vi "RT_control.vi"() -> ()   [LabVIEW 2019]
uses:
  <vilib>/platform/TimedLoop/XDataNode/XDataNode.xnode
  <vilib>/Platform/TimedLoop/XDataNode/nitl_modes.ctl
  <vilib>/Platform/TimedLoop/XDataNode/XDNodeRunTimeDep.lvlib
  <vilib>/Platform/TimedLoop/XDataNode/wakeup.ctl
  <vilib>/Platform/TimedLoop/XDataNode/timing_clust.ctl
  <vilib>/Utility/file.llb/Write Delimited Spreadsheet (DBL).vi
  <vilib>/myRIO/Instrument Drivers/Onboard IO/PWM/PWM.lvlib
  <vilib>/Utility/Variable/NI_VariableUtilities.lvlib
  <vilib>/myRIO/Express VI/IRQ/IRQ Express VI.xnode
  rpm.vi
  <vilib>/myRIO/Instrument Drivers/IRQ/IO IRQ/IO IRQ.lvlib
  <vilib>/myRIO/Common/Instrument Driver Framework/myRIO v1.0/IRQ/typedefs/DI IRQ Type.ctl
  ISR.vi
  <vilib>/myRIO/Common/Instrument Driver Framework/myRIO v1.0/IRQ/typedefs/Callback VI Ref.ctl
  <vilib>/myRIO/Instrument Drivers/IRQ/IO IRQ/vis/myRIO Register DI IRQ.xnode
  <vilib>/myRIO/Common/Instrument Driver Framework/myRIO v1.0/IRQ/vis/myRIO v1.1 Register DI IRQ.vi
  <vilib>/userDefined/High Color/nirio_resource_hc.ctl
  <vilib>/Analysis/NI_AALBase.lvlib
panel:
  out "tf":dbl
  out "fs":dbl
  out "N":i32
  out "i":i32
  out "Max. Iteration Duration":i64
  out "error out (no error) 2":errorcluster
  out "Iteration Duration":i64
  out "omega_vec":dbl[](array[numeric])
  out "Interrupt On":bool
  in  "RPM Inst Data":path=path "/tmp/log.csv"
  out "Omega":dbl[](graph)
  in  "error in (no error)":errorcluster
  out "Np":dbl
  out "ft":dbl
  in  "Input Data":path=path "/tmp/log.csv"
  out "Finished late":bool
  out "Acquisition State":bool
  in  "Run Time (s)":dbl
  in  "Sampling \nFrequency (Hz)":dbl
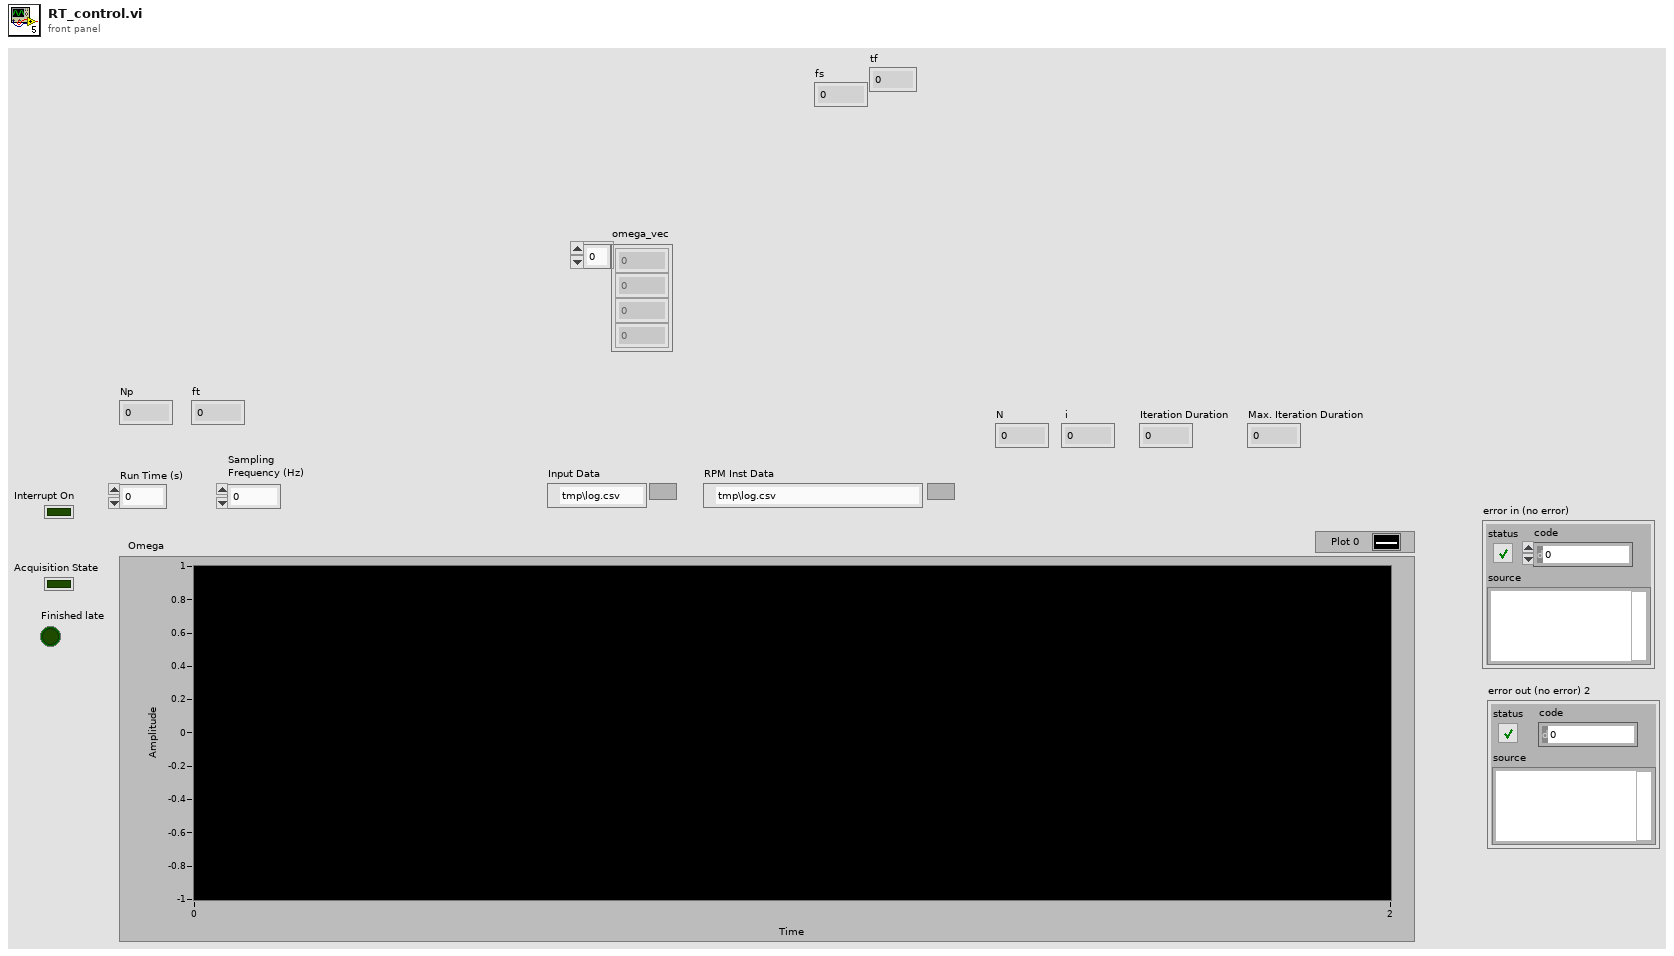
[diagram p1: front panel]
types:
  T1 = typedef "PWM.lvlib/PWM Reference.ctl" = cluster{"myRIO Reference":T2, "PWM Channels Enum":T6, "PWM Configuration":T7}
  T2 = typedef "myRIO Generic Hardware Reference.ctl" = cluster{"myRIO Model":T3, "myRIO Hardware Reference":T4}
  T3 = typedef "Hardware Version Enum.ctl" = enum16{"Unknown", "myRIO-1900", "myRIO-1950", "roboRIO", "NI ELVIS RIO CM", "ELVIS III"}
  T4 = typedef "myRIO v1.0 Reference.ctl" = cluster{"Generic FPGA Reference":T5, "Allow multiple opens":bool}
  T5 = typedef "Generic FPGA Reference.ctl" = refnum<k20>
  T6 = typedef "PWM Channels Enum.ctl" = enum16{"Not Connected", "C/PWM0", "C/PWM1", "A/PWM0", "A/PWM1", "A/PWM2", "A/PWM3", "A/PWM4", "A/PWM5", "A/PWM6", "A/PWM7", "A/PWM8", "A/PWM9", "A/PWM10", "A/PWM11", "A/PWM12", "A/PWM13", "A/PWM14", "A/PWM15", "A/PWM16", "A/PWM17", "A/PWM18", "A/PWM19", "B/PWM0", "B/PWM1", "B/PWM2", "B/PWM3", "B/PWM4", "B/PWM5", "B/PWM6", "B/PWM7", "B/PWM8", "B/PWM9", "B/PWM10", "B/PWM11", "B/PWM12", "B/PWM13", "B/PWM14", "B/PWM15", "B/PWM16", "B/PWM17", "B/PWM18", "B/PWM19", "PWM/PWM0", "PWM/PWM1", "PWM/PWM2", "PWM/PWM3", "PWM/PWM4", "PWM/PWM5", "PWM/PWM6", "PWM/PWM7", "PWM/PWM8", "PWM/PWM9"}
  T7 = typedef "PWM.lvlib/PWM Configuration.ctl" = cluster{"Frequency":dbl, "Duty Cycle":dbl}
  T8 = typedef "XDNodeRunTimeDep.lvlib/timing_clust.ctl" = cluster{"Expected End [f-1]":u64, "Actual End [f-1]":u64, "Finished Late? [f-1]":bool, "Expected End [i-1]":u64, "Actual End [i-1]":u64, "Finished Late? [i-1]":bool, "Expected Start [i]":u64, "Actual Start [i]":u64, "Expected Start [f]":u64, "Actual Start [f]":u64, "Source Name":string, "Structure Name":string, "Period":i64, "Deadline":i64, "Offset":i64, "Start":i64, "Priority":i32, "Timeout":i32, "Mode":T9, "Wakeup Reason":T10, "Error":errorcluster, "Source Type":string, "Secondary Source Type":string, "Global End Time":u64, "Global Start Time":u64, "Frame Duration":u64, "Iteration Duration":u64, "Assigned CPU":i32, "I/O Scan Engine Mode":u32}
  T9 = typedef "XDNodeRunTimeDep.lvlib/nitl_modes.ctl" = enum32{"No Change", "Process missed periods, maintain original phase", "Discard missed periods, maintain original phase", "Process missed periods, ignore original phase", "Discard missed periods, ignore original phase"}
  T10 = typedef "XDNodeRunTimeDep.lvlib/wakeup.ctl" = enum32{"Normal", "Aborted", "Asynchronous wakeup", "Timing source error", "Timed loop error", "Timeout"}
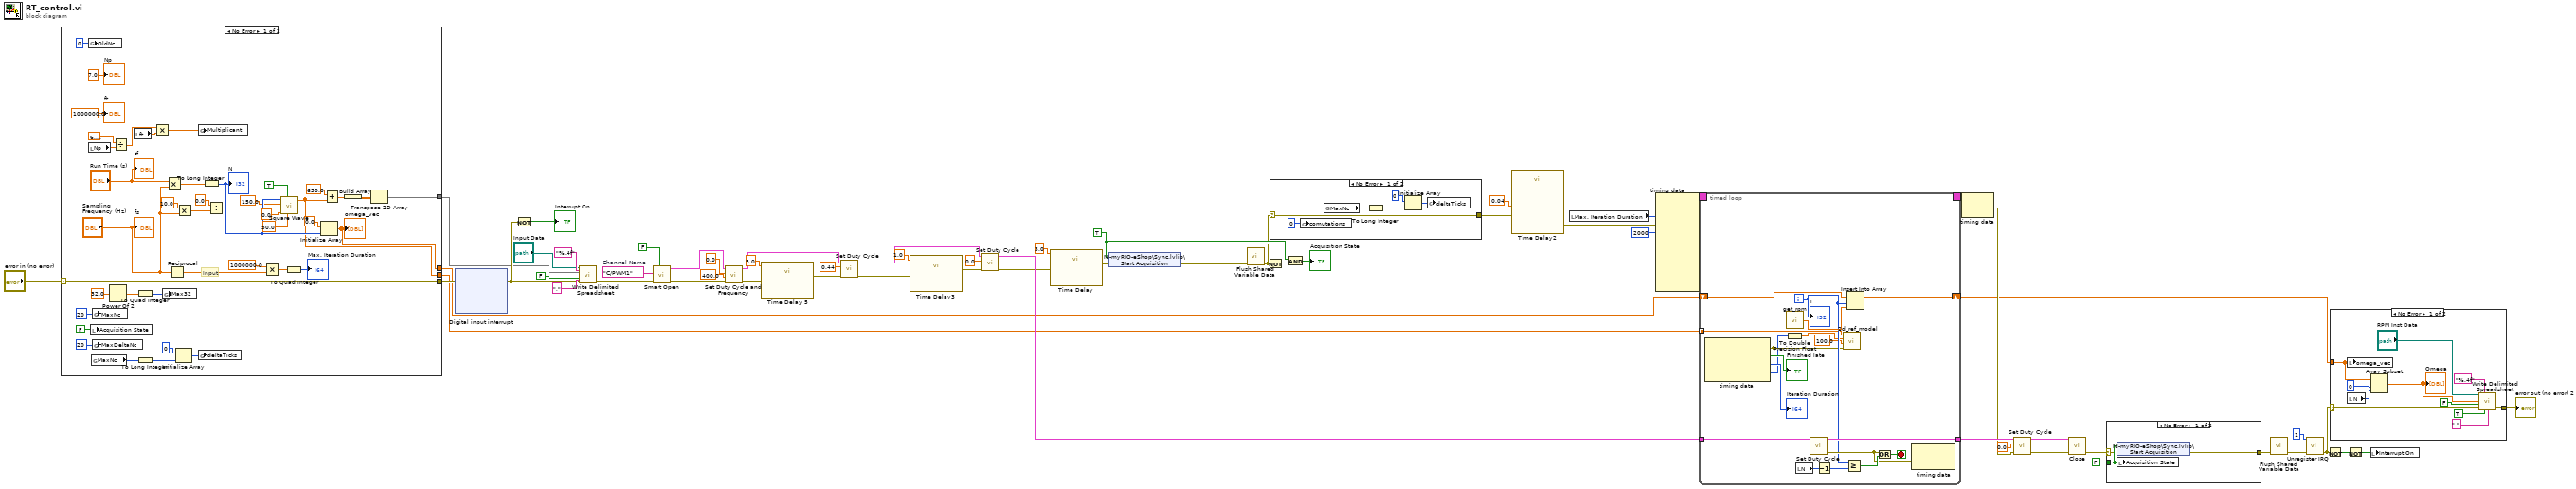
[diagram p0: block diagram]
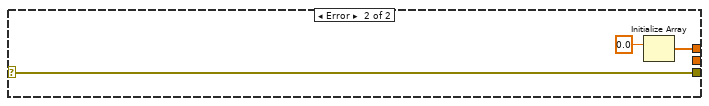
[diagram p5: hidden frame]
diagram:
  w54 = tag "C/PWM1"  # Channel Name
  w37 = TRUE ("Acquisition State")
  n1 = case shown="No Error" "error in (no error)" {
    selector: "error in (no error)" -> [w98 w104]
    tunnel: [w98 w104] -> w34
    tunnel: [w81 w102] -> w9
    tunnel: [w79 _] -> w2
    tunnel: [w60 _] -> w1
    frame No Error {
      # "Input"
      n2 = local read "Np"() -> (w94:dbl)
      n3 = global write "rpm.vi" "OldNc"(i64 0 ("MaxNc")) -> ()
      n4 = local write "Acquisition State"(FALSE ("Acquisition State")) -> ()
      n5 = global read "rpm.vi" "MaxNc"() -> (w83:i64)
      n6 = global write "rpm.vi" "MaxNc"(i64 20 ("MaxNc")) -> ()
      n7 = global write "rpm.vi" "MaxDeltaNc"(i64 20 ("MaxDeltaNc")) -> ()
      n8 = Power Of 2(x=32.0) -> (2^x=w100:dbl)
      n9 = Divide(x=6.283185307179586, y=w94) -> (x/y=w93:dbl)
      n10 = local read "ft"() -> (w92:dbl)
      n11 = To Quad Integer(1:w100) -> (0:w91:i64)
      n12 = To Long Integer(number=w83) -> (32bit integer=w82:i32)
      n13 = Multiply(x=w93, y=w92) -> (x*y=w101:dbl)
      n14 = global write "rpm.vi" "Max32"(w91) -> ()
      n15 = Multiply(x="Run Time (s)", y="Sampling \nFrequency (Hz)") -> (x*y=w75:dbl)
      n16 = Reciprocal(x="Sampling \nFrequency (Hz)") -> (1/x=w78:dbl)
      n17 = Initialize Array(i64 0, w82) -> (w84:i64[])
      n18 = Multiply(x=10.0, y="Sampling \nFrequency (Hz)") -> (x*y=w63:dbl)
      n19 = global write "rpm.vi" "Multiplicant"(w101) -> ()
      n20 = global write "rpm.vi" "deltaTicks"(w84) -> ()
      n21 = To Long Integer(number=w75) -> (32bit integer=w72:i32)
      "N" <- w72
      n22 = Divide(x=0.0, y=w63) -> (x/y=w65:dbl)
      n23 = Multiply(x=1000000.0, y=w78) -> (x*y=w76:dbl)
      n24 = call <vilib>:"Square Wave.vi"("samples"=w72, "reset phase"=TRUE, "amplitude"=150.0, "frequency"=w65, "duty cycle (%)"=50.0, "phase in"=0.0) -> ("square wave"=w60:dbl[])  [unwired: 2 out]
      n25 = To Quad Integer(1:w76) -> (0:→"Max. Iteration Duration":i64)
      n26 = Initialize Array(0.0 ("element"), w72) -> (w81:dbl[])
      "omega_vec" <- w81
      n27 = Add(x=650.0, y=w60) -> (x+y=w67:dbl[])
      n28 = Build Array(w67) -> (w80:dbl[][])
      n29 = Transpose 2D Array(2D array=w80) -> (transposed array=w79:dbl[][])
      "Np" <- 7.0 ("Numeric")
      "ft" <- 1000000.0 ("ft")
      "fs" <- "Sampling \nFrequency (Hz)"
      "tf" <- "Run Time (s)"
    }
    frame Error {
      n30 = Initialize Array(0.0 ("element")) -> (w102:dbl[])  [unwired: 1 in]
    }
  }
  n31 = xnode "Digital input interrupt"("error in (no error)"=w34) -> ("error out"=w29:errorcluster)
  n32 = Not(x=w29) -> (.not. x?=→"Interrupt On":bool)
  n33 = call-poly <vilib>:"Write Delimited Spreadsheet.vi"("file path (dialog if empty)"="Input Data", "format (%.3f)"="%.4f", "2D data"=w2, "append to file? (new file:F)"=FALSE, "error in (no error)"=w29, "delimiter (\\t)"="," ("delimiter (\\t)")) -> ("error out"=w50:errorcluster)  [unwired: 8 in, 1 out]
  n34 = call <vilib>:"Smart Open.vi"("Allow multiple opens?"=FALSE, "error in (no error)"=w50, "Channel Name"=w54) -> ("error out"=w52:errorcluster, "PWM Ref Out"=w53:T1)  [unwired: 7 in]
  n35 = call <vilib>:"Set Duty Cycle and Frequency.vi"("error in (no error)"=w52, "Frequency [Hz]"=400.0, "Duty Cycle"=0.0, "PWM Ref In"=w53) -> ("error out"=w27:errorcluster, "PWM Ref Out"=w17:T1)  [unwired: 5 in]
  n36 = call "Time Delay 5"("error in (no error)"=w27, "Delay Time (s)"=5.0) -> ("error out"=w18:errorcluster)  [unwired: 9 in]
  n37 = call <vilib>:"Set Duty Cycle.vi"("error in (no error)"=w18, "Duty Cycle"=0.44, "PWM Ref In"=w17) -> ("error out"=w21:errorcluster, "PWM Ref Out"=w15:T1)  [unwired: 6 in]
  n38 = call "Time Delay3"("error in (no error)"=w21, "Delay Time (s)"=1.0) -> ("error out"=w16:errorcluster)  [unwired: 9 in]
  n39 = call <vilib>:"Set Duty Cycle.vi"("error in (no error)"=w16, "Duty Cycle"=0.0, "PWM Ref In"=w15) -> ("error out"=w25:errorcluster, "PWM Ref Out"=w26:T1)  [unwired: 6 in]
  n40 = call "Time Delay"("error in (no error)"=w25, "Delay Time (s)"=3.0) -> ("error out"=w45:errorcluster)  [unwired: 9 in]
  n41 = shared-variable "NI-myRIO-eShop\\Sync.lvlib\\Start Acquisition"(w37, error in=w45) -> (error out=w49:errorcluster)
  n42 = call <vilib>:"Flush Shared Variable Data.vi"("error in (no error)"=w49) -> ("error out"=w23:errorcluster)  [unwired: 10 in]
  n43 = Not(x=w23) -> (.not. x?=w22:bool)
  n44 = case shown="No Error" w23 {
    selector: w23 -> [w109 w111]
    tunnel: [w109 w111] -> w31
    frame No Error {
      n45 = global write "rpm.vi" "comutations"(i64 0 ("comutations")) -> ()
      n46 = global read "rpm.vi" "MaxNc"() -> (w106:i64)
      n47 = To Long Integer(number=w106) -> (32bit integer=w105:i32)
      n48 = Initialize Array(i64 0, w105) -> (w107:i64[])
      n49 = global write "rpm.vi" "deltaTicks"(w107) -> ()
    }
    frame Error {
    }
  }
  n50 = And(x=w37, y=w22) -> (x .and. y?=→"Acquisition State":bool)
  n51 = call "Time Delay2"("error in (no error)"=w31, "Delay Time (s)"=0.04) -> ("error out"=w43:errorcluster)  [unwired: 9 in]
  n52 = local read "Max. Iteration Duration"() -> (w3:i64)
  n53 = node-c288(w3, w43, 2000 ("Priority")) -> (w59:T8)  [unwired: 7 in]
  n54 = timed-loop {
    timing: w59 -> [_]
    timing-out: [_] -> w58
    tunnel: w26 -> [w129]
    tunnel: [w126] -> w40
    shift-right: [w123] -> w10
    shift-left: w9 -> [w124]
    tunnel: w1 -> [w117] mode=indexing
    i -> [w120]
    stop <- w128 stop-if-true
    n55 = node-c288() -> (w116:errorcluster, →"Finished late":bool, →"Iteration Duration":i64, w113:i64)  [unwired: 1 in]
    n56 = call "get_rpm.vi"("error in (no error)"=w116) -> ("RPM"=w125:dbl)  [unwired: 1 out]
    n57 = To Double Precision Float(number=w113) -> (double precision float=w114:dbl)
    n58 = local read "N"() -> (w118:i32)
    n59 = call <vilib>:"Set Duty Cycle.vi"("PWM Ref In"=w129) -> ("error out"=w121:errorcluster, "PWM Ref Out"=w126:T1)  [unwired: 8 in]
    n60 = Decrement(x=w118) -> (x-1=w122:i32)
    n61 = call "2d_ref_model.vi"("error in (no error)"=w116, "f_band"=100.0, "dt"=w114, "x"=w117) -> ()  [unwired: 1 in, 2 out]
    n62 = Greater Or Equal?(x=w120, y=w122) -> (x >= y?=w127:bool)
    n63 = Insert Into Array(array=w124, index=w120, new element=w125) -> (w123:dbl[])
    n64 = Or(x=w121, y=w127) -> (x .or. y?=w128:bool)
    n65 = node-c288(w121) -> ()  [unwired: 1 in, 1 out]
    "i" <- w120
  }
  n66 = node-c288(w58) -> (w39:errorcluster)
  n67 = call <vilib>:"Set Duty Cycle.vi"("error in (no error)"=w39, "Duty Cycle"=0.0, "PWM Ref In"=w40) -> ("error out"=w7:errorcluster, "PWM Ref Out"=w8:T1)  [unwired: 6 in]
  n68 = call <vilib>:"Close.vi"("error in (no error)"=w7, "PWM Ref In"=w8) -> ("error out"=w6:errorcluster)  [unwired: 9 in]
  n69 = case shown="No Error" w6 {
    selector: w6 -> [w138 w141]
    tunnel: [w140 w141] -> w48
    tunnel: FALSE ("Start Acquisition") -> [w139 _]
    frame No Error {
      n70 = shared-variable "NI-myRIO-eShop\\Sync.lvlib\\Start Acquisition"(w139, error in=w138) -> (error out=w140:errorcluster)
      n71 = local write "Acquisition State"(w139) -> ()
    }
    frame Error {
    }
  }
  n72 = call <vilib>:"Flush Shared Variable Data.vi"("error in (no error)"=w48) -> ("error out"=w32:errorcluster)  [unwired: 10 in]
  n73 = call <vilib>:"Unregister IRQ.vi"("error in (no error)"=w32, "IRQ Number"=u8 1) -> ("error out"=w12:errorcluster)  [unwired: 9 in]
  n74 = Not(x=w12) -> (.not. x?=w14:bool)
  n75 = case shown="No Error" w12 {
    selector: w12 -> [w147 w153]
    tunnel: [w146 w153] -> w11
    tunnel: w10 -> [w143 _]
    frame No Error {
      n76 = local write "omega_vec"(w143) -> ()
      n77 = local read "N"() -> (w142:i32)
      n78 = Array Subset(array=w143, index=0, length=w142) -> (w145:dbl[])
      "Omega" <- w145
      n79 = call-poly <vilib>:"Write Delimited Spreadsheet.vi"("file path (dialog if empty)"="RPM Inst Data", "format (%.3f)"="%.4f", "1D data"=w145, "append to file? (new file:F)"=FALSE, "error in (no error)"=w147, "transpose? (no:F)"=TRUE, "delimiter (\\t)"="," ("delimiter (\\t)")) -> ("error out"=w146:errorcluster)  [unwired: 7 in, 1 out]
    }
    frame Error {
    }
  }
  "error out (no error) 2" <- w11
  n80 = Not(x=w14) -> (.not. x?=w13:bool)
  n81 = local write "Interrupt On"(w13) -> ()
